vi "application.vi"() -> ()   [LabVIEW 2014, in "application.lvclass"]
uses:
  application.lvclass
  application.lvclass/application.ctl
  <vilib>/Utility/config.llb/NI_LVConfig.lvlib
panel:
  in  "Tab Control":enum32{"Main", "Settings"}(tab)
  in  "Settings":bool
  out "CMD":string caption="命令行"
  in  "file path":path=path "D:/Projects/Personal/Multi-LabVIEW-Selector/Multi-LabVIEW Selector.lvproj" caption="打开文件路径"
  in  "LabVIEW List":string(combo)
  in  "OK":bool
  in  "Cancel":bool
  in  "associate file extension":bool
  in  "System Array":string[](array[string]) caption="File Extension"
  in  "Display Time(ms)":i32 min=0 max=10000 step=100
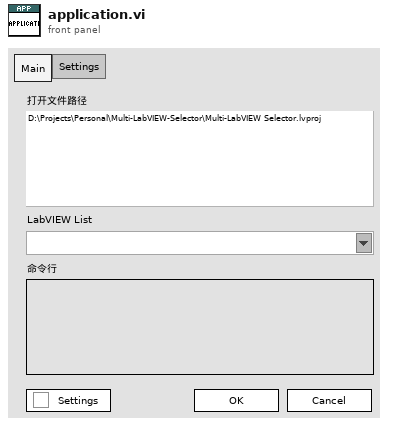
[diagram p1: front panel]
types:
  T1 = enum32{"invalid app kind", "Development System", "Run Time System", "Student Edition", "Embedded LabVIEW", "Evaluation", "Custom"}
  T2 = enum32{"Invalid", "Standard", "Closed", "Hidden", "Minimized", "Maximized"}
  T3 = cluster{"Core":cluster{"Current VI Reference":refnum<vi>, "Close Panel on Exit?":bool}, "RuntimeEngine":bool, "ConfigFilePath":path}
  T4 = cluster{"Current VI Reference":refnum<vi>, "Close Panel on Exit?":bool}
  T5 = typedef "NI_LVConfig.lvlib/Config Data RefNum.ctl" = refnum<k1>
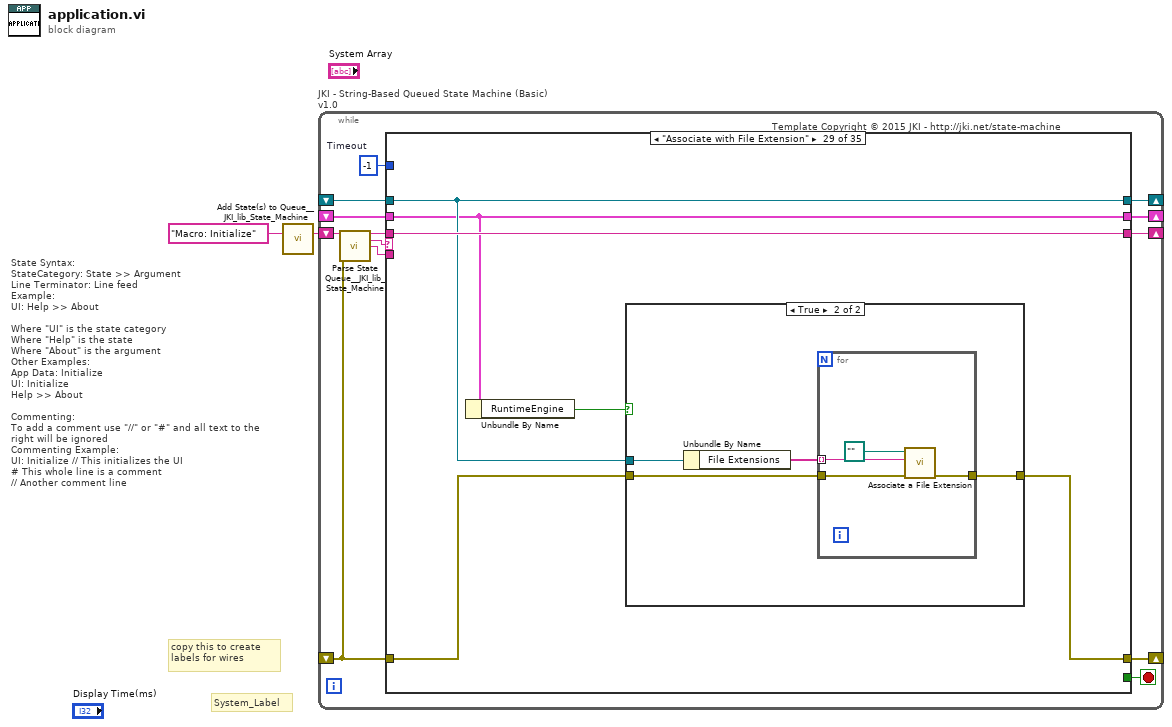
[diagram p0: block diagram]
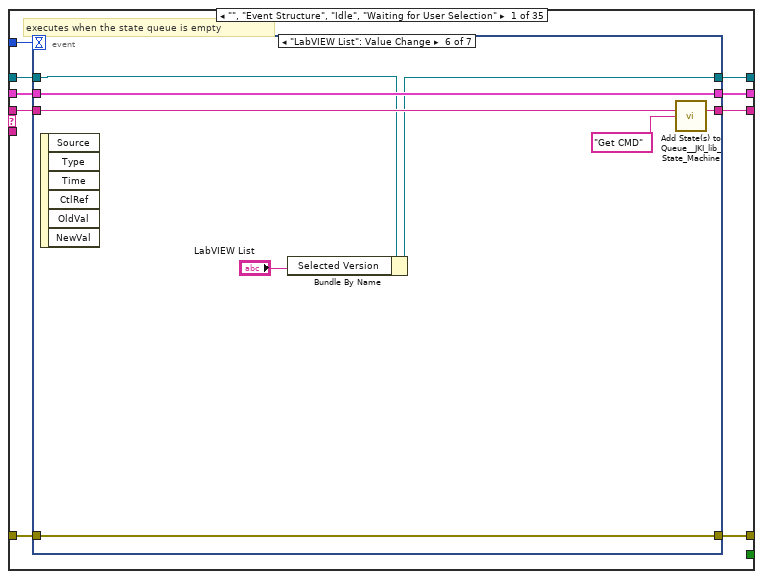
[diagram p2: hidden frame]
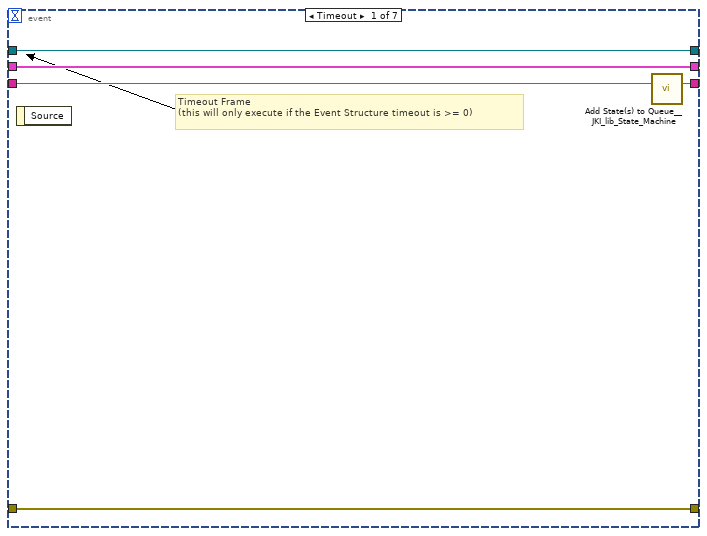
[diagram p3: hidden frame]
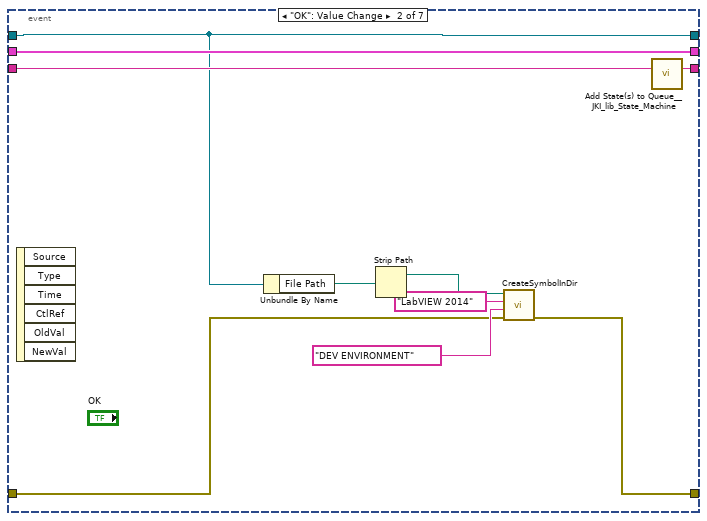
[diagram p4: hidden frame]
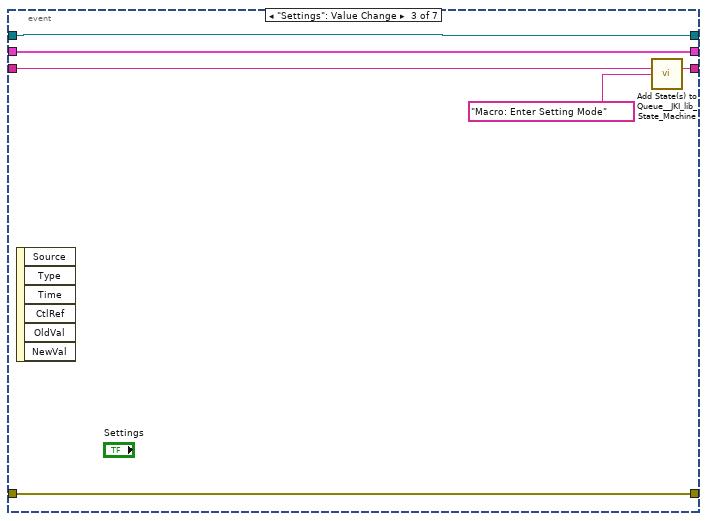
[diagram p5: hidden frame]
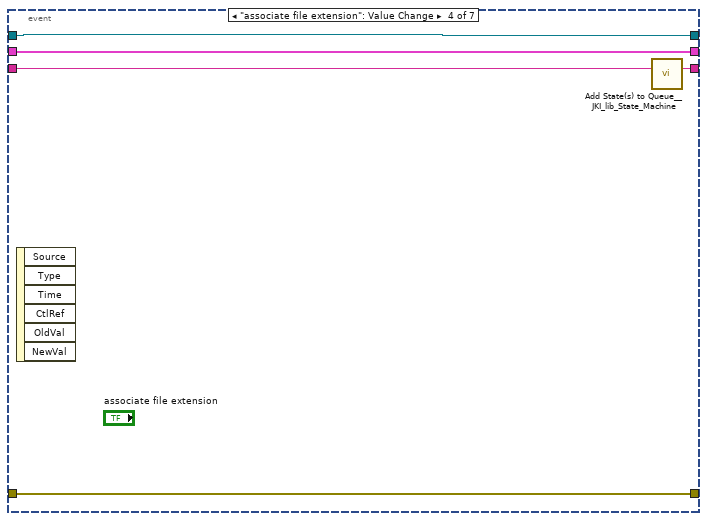
[diagram p6: hidden frame]
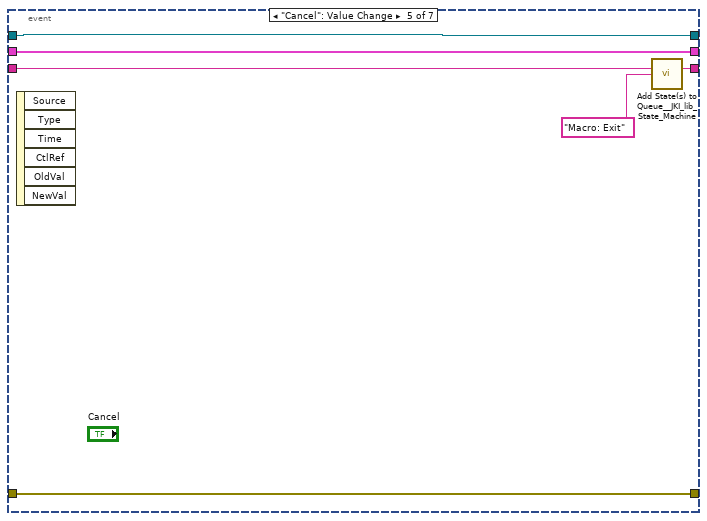
[diagram p7: hidden frame]
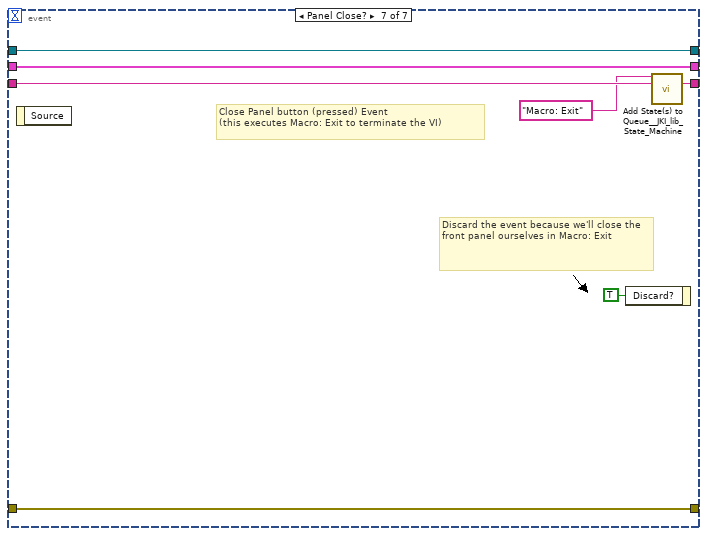
[diagram p8: hidden frame]
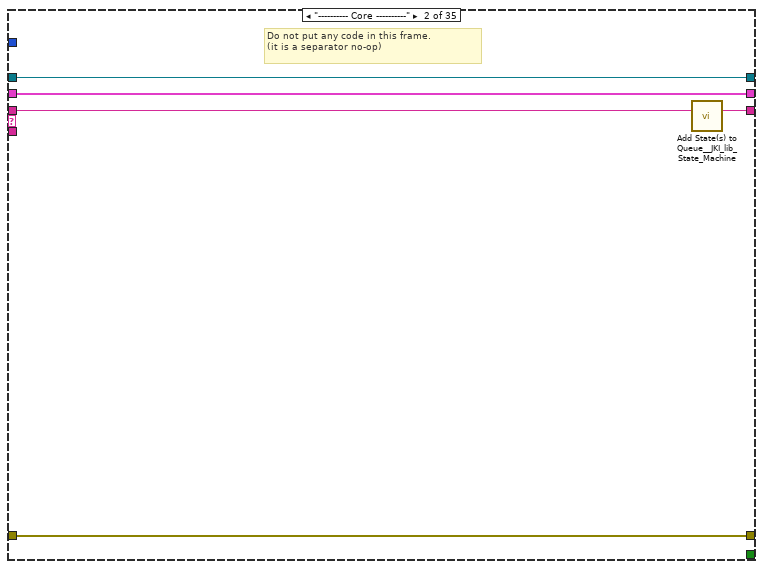
[diagram p9: hidden frame]
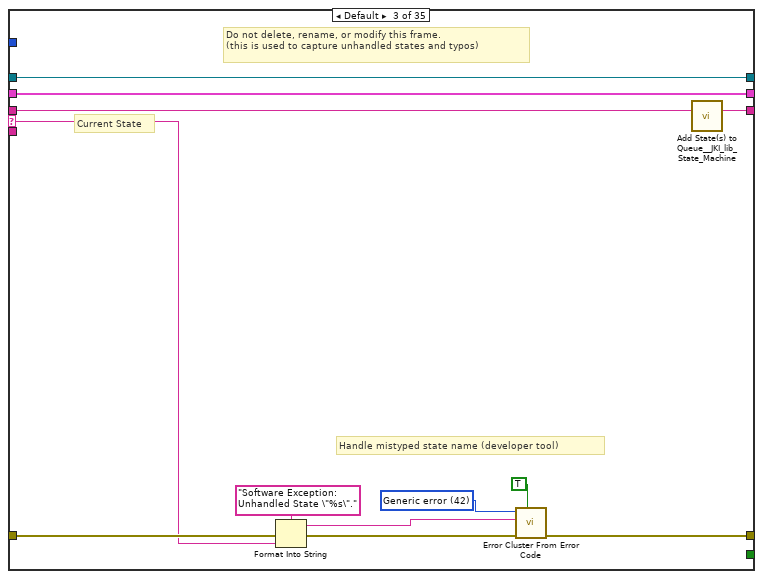
[diagram p10: hidden frame]
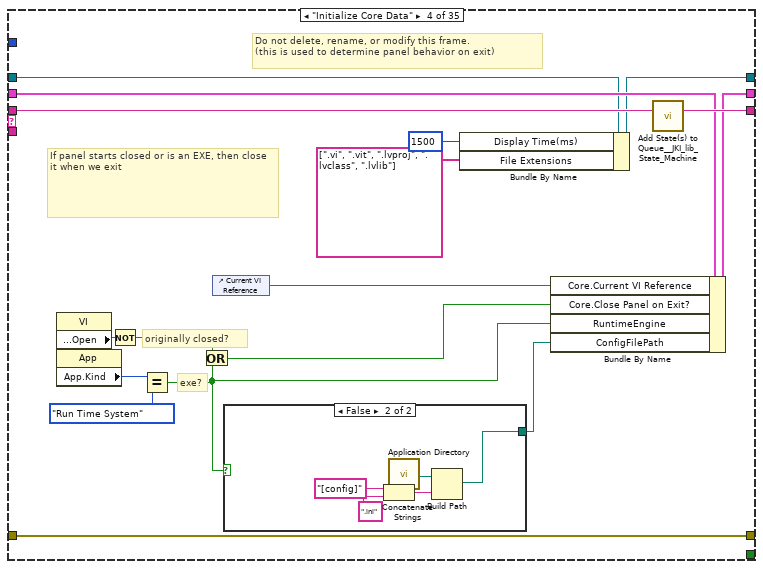
[diagram p11: hidden frame]
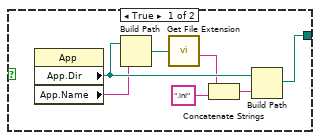
[diagram p12: hidden frame]
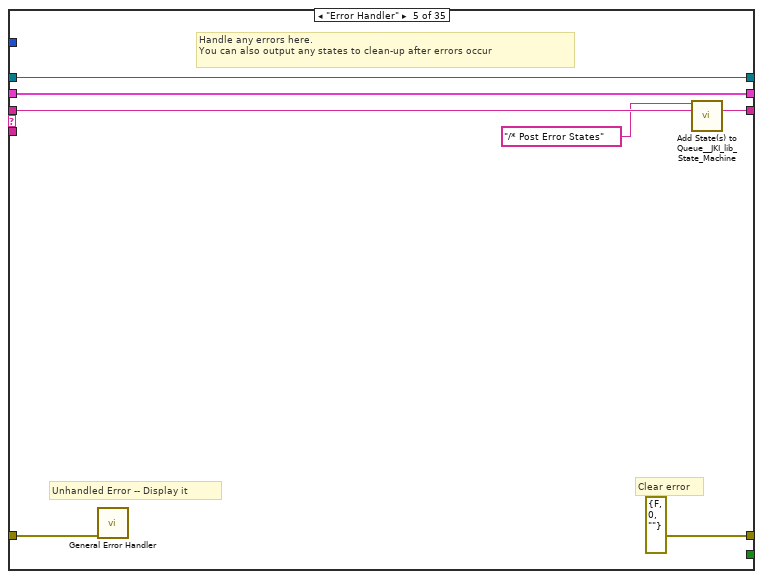
[diagram p13: hidden frame]
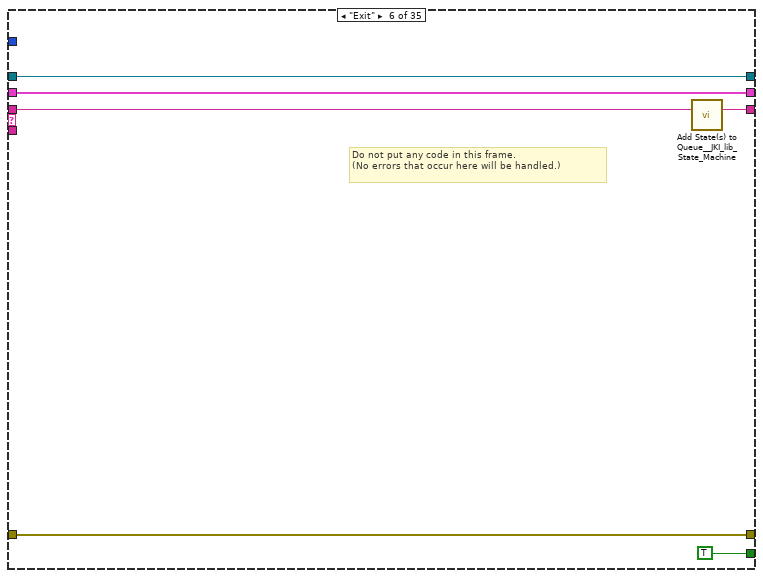
[diagram p14: hidden frame]
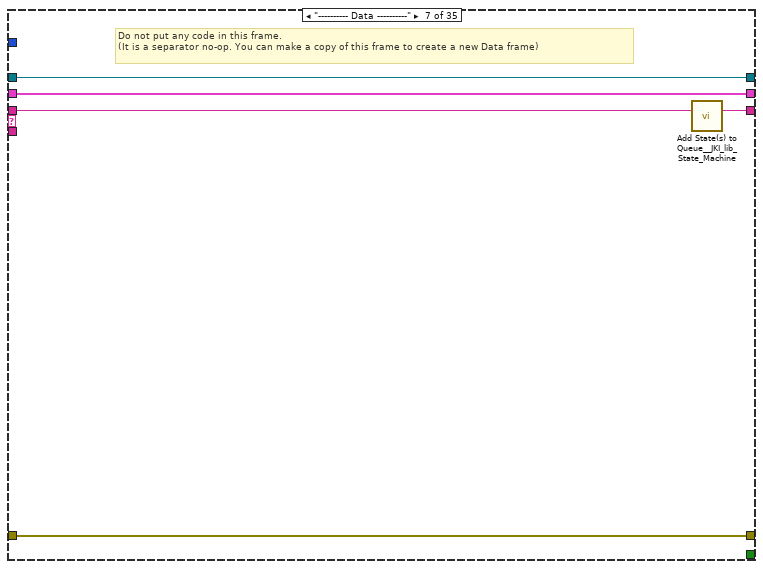
[diagram p15: hidden frame]
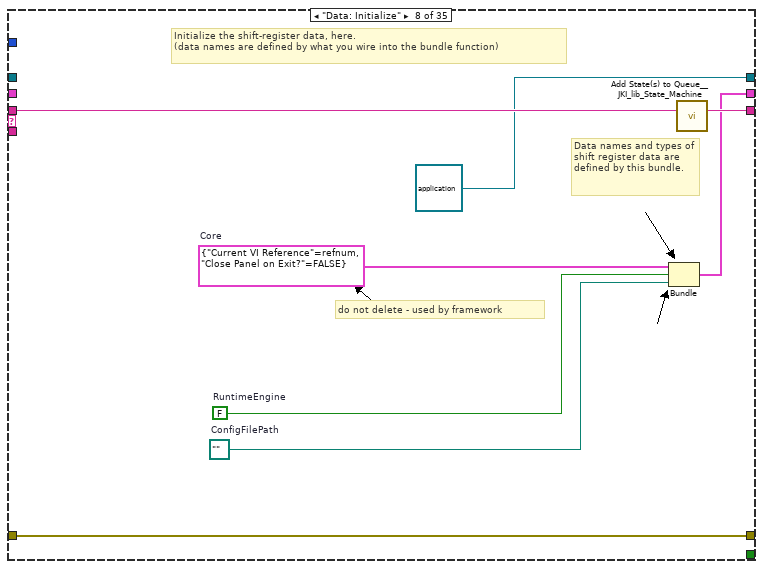
[diagram p16: hidden frame]
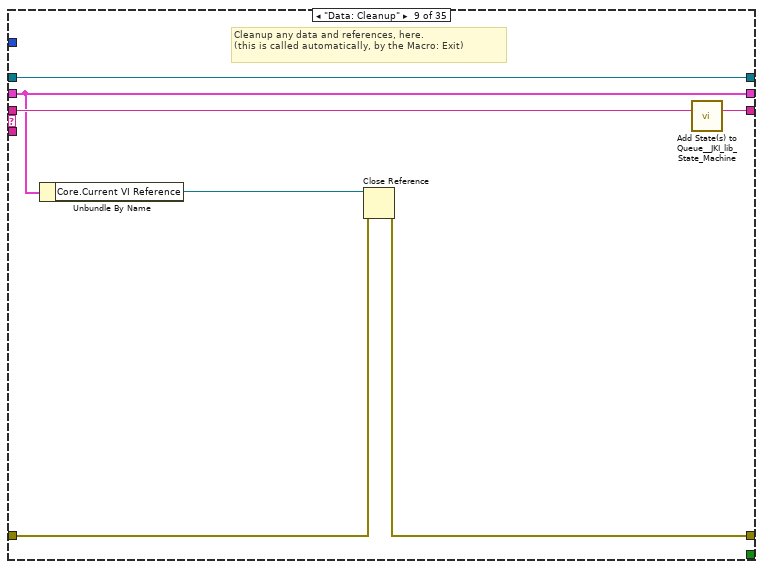
[diagram p17: hidden frame]
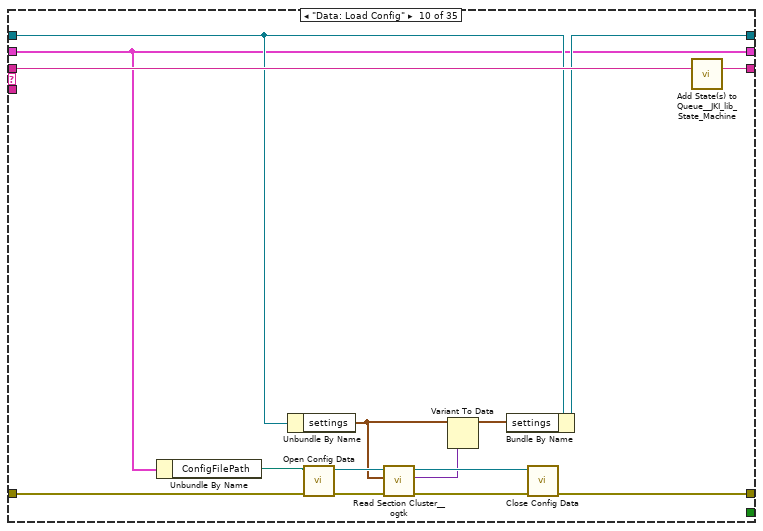
[diagram p18: hidden frame]
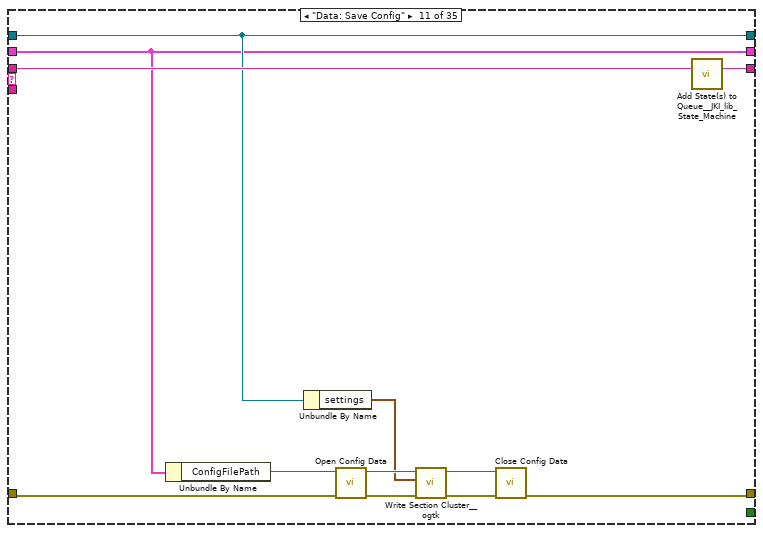
[diagram p19: hidden frame]
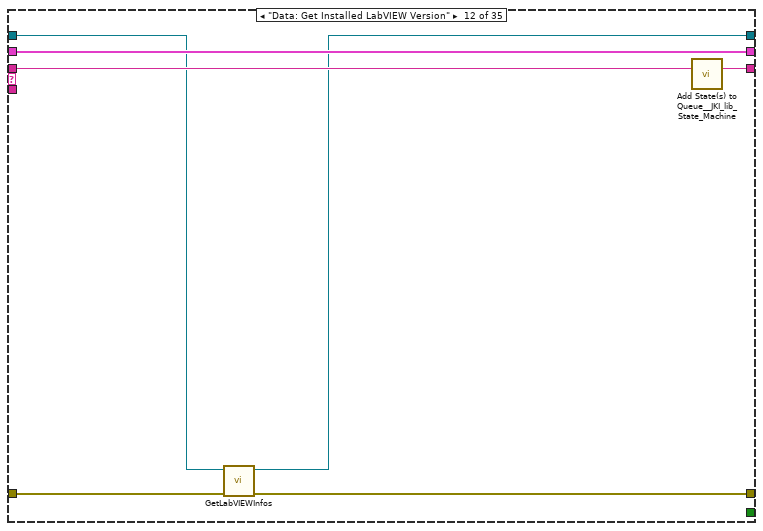
[diagram p20: hidden frame]
diagram:
  # "State Syntax:\nStateCategory: State >> Argument\nLine Terminator: Line feed\nExample:\nUI: Help >> About\n\nWhere \"UI\" is the state category\nWhere \"Help\" is the state\nWhere \"About\" is the argument\nOther Examples:\nApp Data: Initialize\nUI: Initialize\nHelp >> About\n\nCommenting:\nTo add a comment use \"//\" or \"#\" and all text to the right will be ignored\nCommenting Example:\nUI: Initialize // This initializes the UI\n# This whole line is a comment\n// Another comment line"
  # "copy this to create labels for wires"
  # "System_Label"
  n1 = call <vilib>:"Add State(s) to Queue__JKI_lib_State_Machine.vi"("State(s) in (\"\")"="Macro: Initialize") -> ("States Out"=w2:string)  [unwired: 14 in]
  n2 = while "JKI - String-Based Queued State Machine (Basic) v1.0" {
    shift-right: [w8] -> _
    shift-left: _ -> [w7]
    shift-right: [w11] -> _
    shift-left: _ -> [w5]
    shift-right: [w10] -> _
    shift-left: w2 -> [w12]
    shift-right: [w4] -> _
    shift-left: _ -> [w3]
    stop <- w9 stop-if-true
    w6 = -1  # Timeout
    # "Template Copyright © 2015 JKI - http://jki.net/state-machine"
    n3 = call <vilib>:"Parse State Queue__JKI_lib_State_Machine.vi"("State Queue"=w12, "Error In (no error)"=w5) -> ("Remaining States"=w14:string, "Current State"=w15:string, "Arguments"=w13:string)  [unwired: 11 in]
    n4 = case shown="\"Associate with File Extension\"" w15 {
      selector: w15 -> [_ _ w78 _ _ _ _ _ _ _ _ _ _ _ _ _ _ _ _ _ _ _ _ _ _ _ _ _ _ _ _ _ _ _ _]
      tunnel: w14 -> [w24 w76 w82 w105 w124 w130 w135 w143 w150 w165 w177 w184 w189 w200 w211 w223 w251 w259 w266 w273 w280 w286 w297 w303 w309 w314 w322 w325 w336 w350 w359 w383 w396 w408 w417]
      tunnel: w13 -> [_ _ _ _ _ _ _ _ _ _ _ _ _ _ w206 w217 _ _ _ w268 _ _ _ _ _ _ _ _ _ _ _ _ _ _ _]
      tunnel: w7 -> [w22 w73 w80 w97 w121 w128 w132 _ w145 w152 w166 w182 w186 w198 w209 w219 w248 w256 w263 w270 w277 w283 w294 w300 w306 w311 w320 w326 w332 w347 w355 w385 w398 w410 w419]
      tunnel: [w21 w74 w84 w102 errorcluster {"status"=FALSE, "code"=0, "source"=""} ("error out") w127 w133 w140 w146 w157 w170 w180 w187 w196 w207 w220 w249 w257 w264 w271 w278 w284 w295 w301 w307 w312 w318 w323 w334 w348 w361 w373 w386 w399 w416] -> w11
      tunnel: w5 -> [w20 w74 w83 w102 w120 w127 w133 w140 w147 w158 w169 w181 w187 w194 w208 w221 w249 w257 w264 w271 w278 w284 w295 w301 w307 w312 w319 w324 w335 w348 w362 w374 w387 w400 w416]
      tunnel: [w23 w75 w81 w104 w123 w129 w134 w142 w149 w164 w176 w183 w188 w199 w210 w222 w250 w258 w265 w272 w279 w285 w296 w302 w308 w313 w321 w325 w336 w349 w360 w384 w397 w409 w418] -> w10
      tunnel: [_ _ _ _ _ TRUE _ _ _ _ _ _ _ _ _ _ _ _ _ _ _ _ _ _ _ _ _ _ _ _ _ _ _ _ _] -> w9
      tunnel: [w19 w73 w80 w103 w121 w128 w132 w141 w145 w152 w166 w182 w186 w198 w209 w219 w248 w256 w263 w270 w277 w283 w294 w300 w306 w311 w320 w326 w332 w347 w355 w385 w398 w410 w419] -> w8
      tunnel: w6 -> [w18 _ _ _ _ _ _ _ _ _ _ _ _ _ _ _ _ _ _ _ _ _ _ _ _ _ _ _ _ _ _ _ _ _ _]
      tunnel: [w16 w72 w77 w93 w118 w125 w131 refnum<class "application.lvclass"> refnum ("application.lvclass") w144 w156 w168 w178 w185 w197 w205 w216 w247 w253 w262 w269 w276 w281 w287 w299 w305 w310 w316 w327 w333 w346 w358 w375 w388 w401 w411] -> w4
      tunnel: w3 -> [w17 w72 w77 w94 w118 w125 w131 _ w144 w163 w168 w179 w185 w197 w205 w216 w247 w253 w262 w269 w276 w281 w287 w299 w305 w310 w317 w327 w333 w346 w363 w376 w389 w401 w412]
      frame "", "Event Structure", "Idle", "Waiting for User Selection" {
        # "executes when the state queue is empty"
        n5 = event shown="[5] \"LabVIEW List\": Value Change" {
          selector: _ -> [_ _ _ _ _ _ _]
          dyn-events: _ -> [_ _ _ _ _ _ _]
          timeout: w18 -> [_ _ _ _ _ _ _]
          tunnel: w24 -> [w29 w39 w45 w50 w56 w64 w71]
          tunnel: [w28 w38 w44 w49 w55 w63 w70] -> w23
          tunnel: w22 -> [w26 w37 w42 w47 w53 w61 w68]
          tunnel: [w27 w31 w43 w48 w54 w62 w69] -> w21
          tunnel: w20 -> [w27 w32 w43 w48 w54 w62 w69]
          tunnel: [w26 w37 w42 w47 w53 w61 w68] -> w19
          tunnel: w17 -> [w25 w33 w41 w46 w52 w60 w65]
          tunnel: [w25 w33 w41 w46 w52 w58 w65] -> w16
          event Timeout {
            # "Timeout Frame\n(this will only execute if the Event Structure timeout is >= 0)"
            n6 = event-data() -> ()  [unwired: 1 in, 1 out]
            n7 = call <vilib>:"Add State(s) to Queue__JKI_lib_State_Machine.vi"("State(s) in (\"\")"=w29) -> ("States Out"=w28:string)  [unwired: 14 in]
          }
          event "OK": Value Change {
            n8 = event-data() -> ()  [unwired: 1 in, 6 out]
            n9 = Unbundle By Name(w33) -> ("File Path"=w36:path)
            n10 = Strip Path(path=w36) -> (stripped path=w35:path)  [unwired: 1 out]
            n11 = call "CreateSymbolInDir.vi"("error in"=w32, "prefix"="DEV ENVIRONMENT", "Name"="LabVIEW 2014", "Path"=w35) -> ("error out"=w31:errorcluster)  [unwired: 6 in, 1 out]
            n12 = call <vilib>:"Add State(s) to Queue__JKI_lib_State_Machine.vi"("State(s) in (\"\")"=w39) -> ("States Out"=w38:string)  [unwired: 14 in]
          }
          event "Settings": Value Change {
            n13 = event-data() -> ()  [unwired: 1 in, 6 out]
            n14 = call <vilib>:"Add State(s) to Queue__JKI_lib_State_Machine.vi"("State(s) in (\"\")"=w45, "State(s) at Back (\"\")"="Macro: Enter Setting Mode" ("State(s) at Back (\"\")")) -> ("States Out"=w44:string)  [unwired: 13 in]
          }
          event "associate file extension": Value Change {
            n15 = event-data() -> ()  [unwired: 1 in, 6 out]
            n16 = call <vilib>:"Add State(s) to Queue__JKI_lib_State_Machine.vi"("State(s) in (\"\")"=w50) -> ("States Out"=w49:string)  [unwired: 14 in]
          }
          event "Cancel": Value Change {
            n17 = event-data() -> ()  [unwired: 1 in, 6 out]
            n18 = call <vilib>:"Add State(s) to Queue__JKI_lib_State_Machine.vi"("State(s) in (\"\")"=w56, "State(s) at Back (\"\")"="Macro: Exit" ("State(s) at Back (\"\")")) -> ("States Out"=w55:string)  [unwired: 13 in]
          }
          event "LabVIEW List": Value Change {
            n19 = event-data() -> ()  [unwired: 1 in, 6 out]
            n20 = Bundle By Name(cluster=w60, "Selected Version"="LabVIEW List") -> (w58:refnum<class "application.lvclass">)
            n21 = call <vilib>:"Add State(s) to Queue__JKI_lib_State_Machine.vi"("State(s) in (\"\")"=w64, "State(s) at Back (\"\")"="Get CMD" ("State(s) at Back (\"\")")) -> ("States Out"=w63:string)  [unwired: 13 in]
          }
          event Panel Close? {
            # "Discard the event because we'll close the front panel ourselves in Macro: Exit"
            # "Close Panel button (pressed) Event\n(this executes Macro: Exit to terminate the VI)"
            n22 = event-data() -> ()  [unwired: 1 in, 1 out]
            n23 = event-data("Discard?"=TRUE) -> ()  [unwired: 1 in, 1 out]
            n24 = call <vilib>:"Add State(s) to Queue__JKI_lib_State_Machine.vi"("State(s) in Front (\"\")"="Macro: Exit", "State(s) in (\"\")"=w71) -> ("States Out"=w70:string)  [unwired: 13 in]
          }
        }
      }
      frame "---------- Core ----------" {
        # "Do not put any code in this frame.\n(it is a separator no-op)"
        n25 = call <vilib>:"Add State(s) to Queue__JKI_lib_State_Machine.vi"("State(s) in (\"\")"=w76) -> ("States Out"=w75:string)  [unwired: 14 in]
      }
      frame Default {
        w87 = 42 items=["No error", "Argument error", "Memory is full", "Out of zone", "End of file", "File already open", "Generic file I/O error", "File not found", "File permission error", "Disk is full", "Duplicate path", "Too many files open", "System feature not enabled", "Resource file not found", "Cannot add resource", "Resource not found", "Image not found", "Image memory error", "Pen does not exist", "Config type invalid", "Config token not found", "Config parse error", "Config memory error", "Bad external code format", "Bad external code offset", "External code not present", "Null window", "Destroy window error", "Null menu", "Print aborted", "Bad print record", "Print driver error", "Windows error during printing", "Memory error during printing", "Print dialog error", "Generic print error", "Invalid device refnum", "Device not found", "Device parameter error", "Device unit error", "Cannot open device", "Device call aborted", "Generic error", "Cancelled by user", "Object ID too low", "Object ID too high", "Object not in heap", "Unknown heap", "Unknown object (invalid DefProc)", "Unknown object (DefProc not in table)", "Message out of range", "Invalid (null) method", "Unknown message", "Manager call not supported", "Bad address", "Network operation in progress", "Network operation timed out", "Connection is busy", "Network attribute not supported", "Network error", "Address in use", "System out of memory", "Connection aborted", "Connection refused", "Not connected", "Already connected", "Connection closed", "Initialization error (interapplication manager)", "Bad occurrence", "Wait on unbound occurrence handler", "Occurrence queue overflow", "Datalog type conflict", "Unused", "Unrecognized type (interapplication manager)", "Memory corrupt", "Failed to make temporary DLL", "Old CIN version", "Drag socket not found", "Failed to load drop-object", "Failed to register OLE object", "Failed to release OLE object", "Format specifier type mismatch", "Unknown format specifier", "Too few format specifiers", "Too many format specifiers", "Scan failed", "Newer CIN version", "Error converting to variant", "Runtime menu error", "Password tampered", "Variant attribute not found", "Incompatible variant data type", "Event data is not available", "Event Store is not present", "Occurrence is not found", "Event Queue is not created", "Event info is not available", "Refnum passed is NULL", "Error retrieving Class GUID", "Error retrieving CoClass GUID", "Error retrieving TypeLib GUID.", "Bad built application magic bytes.", "Specific driver is different from the specific driver associated with the Logical Name.", "There is no session opened to the class driver.", "Max Error", "MAX - Error with config objects", "MAX - Error loading configuration", "MAX - Group not supported"]
        # "Current State"
        # "Do not delete, rename, or modify this frame.\n(this is used to capture unhandled states and typos)"
        # "Handle mistyped state name (developer tool)"
        n26 = Format Into String(format string="Software Exception: Unhandled State \"%s\"." ("message"), error in=w83, w78) -> (resulting string=w86:string, error out=w85:errorcluster)  [unwired: 1 in]
        n27 = call <vilib>:"Error Cluster From Error Code.vi"("show call chain? (False)"=TRUE, "error in (no error)"=w85, "error message (\"\")"=w86, "error code (0)"=w87) -> ("error out"=w84:errorcluster)  [unwired: 5 in]
        n28 = call <vilib>:"Add State(s) to Queue__JKI_lib_State_Machine.vi"("State(s) in (\"\")"=w82) -> ("States Out"=w81:string)  [unwired: 14 in]
      }
      frame "Initialize Core Data" {
        # "Do not delete, rename, or modify this frame.\n(this is used to determine panel behavior on exit)"
        # "originally closed?"
        # "exe?"
        # "If panel starts closed or is an EXE, then close it when we exit"
        n29 = property class="VI"() -> ("Front Panel.Open"=w101:bool)  [unwired: 2 in, 2 out]
        n30 = property class="App"() -> ("App.Kind"=w100:T1)  [unwired: 2 in, 2 out]
        n31 = Not(x=w101) -> (.not. x?=w98:bool)
        n32 = Equal?(x=w100, y=T1."Run Time System" ("Application:Kind")) -> (x = y?=w89:bool)
        n33 = Or(x=w98, y=w89) -> (x .or. y?=w96:bool)
        n34 = control-ref of="Current VI Reference"() -> (w95:refnum<vi>)
        n35 = case shown="False" w89 {
          tunnel: [w110 w114] -> w90
          frame True {
            n36 = property class="App"() -> ("App.Dir"=w109:path, "App.Name"=w108:string)  [unwired: 2 in, 2 out]
            n37 = Build Path(base path=w109, name or relative path=w108) -> (appended path=w107:path)
            n38 = call <vilib>:"Get File Extension.vi"("file"=w107) -> ("filename without extension"=w106:string)  [unwired: 7 in, 3 out]
            n39 = Concatenate Strings(w106, ".ini" ("Application:Name")) -> (w111:string)
            n40 = Build Path(base path=w109, name or relative path=w111) -> (appended path=w110:path)
          }
          frame False {
            n41 = Concatenate Strings("[config]" ("string"), ".ini" ("Application:Name")) -> (w115:string)
            n42 = call <vilib>:"Application Directory.vi"() -> ("Application Directory"=w116:path)
            n43 = Build Path(base path=w116, name or relative path=w115) -> (appended path=w114:path)
          }
        }
        n44 = Bundle By Name(cluster=w94, "Display Time(ms)"=1500 ("settings.Display Time(ms)"), "File Extensions"=string[] [".vi", ".vit", ".lvproj", ".lvclass", ".lvlib"]) -> (w93:refnum<class "application.lvclass">)
        n45 = Bundle By Name(cluster=w97, "Core.Current VI Reference"=w95, "Core.Close Panel on Exit?"=w96, "RuntimeEngine"=w89, "ConfigFilePath"=w90) -> (w103:T3)
        n46 = call <vilib>:"Add State(s) to Queue__JKI_lib_State_Machine.vi"("State(s) in (\"\")"=w105) -> ("States Out"=w104:string)  [unwired: 14 in]
      }
      frame "Error Handler" {
        # "Unhandled Error -- Display it"
        # "Handle any errors here.\nYou can also output any states to clean-up after errors occur"
        # "Clear error"
        n47 = call <vilib>:"General Error Handler.vi"("error in (no error)"=w120) -> ()  [unwired: 10 in, 5 out]
        n48 = call <vilib>:"Add State(s) to Queue__JKI_lib_State_Machine.vi"("State(s) in Front (\"\")"="/* Post Error States", "State(s) in (\"\")"=w124) -> ("States Out"=w123:string)  [unwired: 13 in]
      }
      frame "Exit" {
        # "Do not put any code in this frame.\n(No errors that occur here will be handled.)"
        n49 = call <vilib>:"Add State(s) to Queue__JKI_lib_State_Machine.vi"("State(s) in (\"\")"=w130) -> ("States Out"=w129:string)  [unwired: 14 in]
      }
      frame "---------- Data ----------" {
        # "Do not put any code in this frame.\n(It is a separator no-op. You can make a copy of this frame to create a new Data frame)"
        n50 = call <vilib>:"Add State(s) to Queue__JKI_lib_State_Machine.vi"("State(s) in (\"\")"=w135) -> ("States Out"=w134:string)  [unwired: 14 in]
      }
      frame "Data: Initialize" {
        w137 = T4 {"Current VI Reference"=refnum, "Close Panel on Exit?"=FALSE}  # Core
        w139 = FALSE  # RuntimeEngine
        w138 = path ""  # ConfigFilePath
        # "do not delete - used by framework"
        # "Data names and types of shift register data are defined by this bundle."
        # "Initialize the shift-register data, here.\n(data names are defined by what you wire into the bundle function)"
        n51 = Bundle("Core"=w137, "RuntimeEngine"=w139, "ConfigFilePath"=w138) -> (w141:T3)  [unwired: 1 in]
        n52 = call <vilib>:"Add State(s) to Queue__JKI_lib_State_Machine.vi"("State(s) in (\"\")"=w143) -> ("States Out"=w142:string)  [unwired: 14 in]
      }
      frame "Data: Cleanup" {
        # "Cleanup any data and references, here.\n(this is called automatically, by the Macro: Exit)"
        n53 = Unbundle By Name(w145) -> ("Core.Current VI Reference"=w148:refnum<vi>)
        n54 = Close Reference(reference=w148, error in (no error)=w147) -> (error out=w146:errorcluster)
        n55 = call <vilib>:"Add State(s) to Queue__JKI_lib_State_Machine.vi"("State(s) in (\"\")"=w150) -> ("States Out"=w149:string)  [unwired: 14 in]
      }
      frame "Data: Load Config" {
        n56 = Unbundle By Name(w152) -> ("ConfigFilePath"=w151:path)
        n57 = Unbundle By Name(w163) -> ("settings"=w153:cluster{"Display Time(ms)":i32})
        n58 = call <vilib>:"Open Config Data.vi"("error in (no error)"=w158, "configuration file path"=w151) -> ("error out"=w161:errorcluster, "refnum"=w162:T5)  [unwired: 7 in, 1 out]
        n59 = call <userlib>:"Read Section Cluster__ogtk.vi"("error in (no error)"=w161, "Section Formatted Cluster Type"=w153, "refnum"=w162) -> ("error out"=w159:errorcluster, "Section Formatted Cluster"=w154:variant, "dup refnum"=w160:T5)  [unwired: 4 in, 2 out]
        n60 = Variant To Data(type=w153, Variant=w154) -> (data=w155:cluster{"Display Time(ms)":i32})  [unwired: 1 in, 1 out]
        n61 = Bundle By Name(cluster=w163, "settings"=w155) -> (w156:refnum<class "application.lvclass">)
        n62 = call <vilib>:"Close Config Data.vi"("error in (no error)"=w159, "refnum"=w160) -> ("error out"=w157:errorcluster)  [unwired: 8 in, 1 out]
        n63 = call <vilib>:"Add State(s) to Queue__JKI_lib_State_Machine.vi"("State(s) in (\"\")"=w165) -> ("States Out"=w164:string)  [unwired: 14 in]
      }
      frame "Data: Save Config" {
        n64 = Unbundle By Name(w166) -> ("ConfigFilePath"=w167:path)
        n65 = Unbundle By Name(w168) -> ("settings"=w171:cluster{"Display Time(ms)":i32})
        n66 = call <vilib>:"Open Config Data.vi"("error in (no error)"=w169, "configuration file path"=w167) -> ("error out"=w174:errorcluster, "refnum"=w175:T5)  [unwired: 7 in, 1 out]
        n67 = call <userlib>:"Write Section Cluster__ogtk.vi"("error in (no error)"=w174, "Section Formatted Cluster"=w171, "refnum"=w175) -> ("error out"=w172:errorcluster, "dup refnum"=w173:T5)  [unwired: 7 in]
        n68 = call <vilib>:"Close Config Data.vi"("error in (no error)"=w172, "refnum"=w173) -> ("error out"=w170:errorcluster)  [unwired: 8 in, 1 out]
        n69 = call <vilib>:"Add State(s) to Queue__JKI_lib_State_Machine.vi"("State(s) in (\"\")"=w177) -> ("States Out"=w176:string)  [unwired: 14 in]
      }
      frame "Data: Get Installed LabVIEW Version" {
        n70 = call "GetLabVIEWInfos.vi"("error in (no error)"=w181, "application.lvclass"=w179) -> ("error out"=w180:errorcluster, "application.lvclass (dup)"=w178:refnum<class "application.lvclass">)  [unwired: 8 in]
        n71 = call <vilib>:"Add State(s) to Queue__JKI_lib_State_Machine.vi"("State(s) in (\"\")"=w184) -> ("States Out"=w183:string)  [unwired: 14 in]
      }
      frame "---------- UI ----------" {
        # "Do not put any code in this frame.\n(It is a separator no-op. You can make a copy of this frame to create a new UI frame)"
        n72 = call <vilib>:"Add State(s) to Queue__JKI_lib_State_Machine.vi"("State(s) in (\"\")"=w189) -> ("States Out"=w188:string)  [unwired: 14 in]
      }
      frame "UI: Initialize" {
        # "Initialize the User Interface, here.\n(this is called automatically, by the Macro: Init)"
        n73 = disable-structure shown="Default" {
          disable-tunnel: [FALSE ("Tabs Visible?") TRUE ("Tabs Visible?")] -> w192
          disable-tunnel: [w201 w203] -> w191
          disable-tunnel: [w201 w203] -> w190
          frame condition #0 {
            w201 = u32 16777216
          }
          frame condition #1 (active) {
            w203 = u32 16777216
          }
        }
        n74 = property on="Tab Control" class="TabCtl (strict)"(error in=w194, "Tabs Visible?"=w192, "BG Color"=w191, "FG Color"=w190) -> (error out=w193:errorcluster)  [unwired: 1 in, 1 out]
        n75 = call <userlib>:"Fit VI window to Content__ogtk.vi"("error in (no error)"=w193, "border spacing (2 px)"=0) -> ("error out"=w196:errorcluster)  [unwired: 4 in, 1 out]
        n76 = call <vilib>:"Add State(s) to Queue__JKI_lib_State_Machine.vi"("State(s) in (\"\")"=w200) -> ("States Out"=w199:string)  [unwired: 14 in]
      }
      frame "UI: Cursor Set" {
        # "Argument"
        # "Set and Unset Cursor Busy.\n(Usage: \"UI: Cursor Set >> Busy|Idle\")"
        n77 = case shown="\"Idle\", Default" w206 {
          tunnel: w208 -> [w213 w215]
          tunnel: [w212 w214] -> w207
          frame "Idle", Default {
            n78 = call <vilib>:"Unset Busy.vi"("error in (no error)"=w213) -> ("error out"=w212:errorcluster)  [unwired: 10 in]
          }
          frame "Busy" {
            n79 = call <vilib>:"Set Busy.vi"("error in (no error)"=w215) -> ("error out"=w214:errorcluster)  [unwired: 9 in, 1 out]
          }
        }
        n80 = call <vilib>:"Add State(s) to Queue__JKI_lib_State_Machine.vi"("State(s) in (\"\")"=w211) -> ("States Out"=w210:string)  [unwired: 14 in]
      }
      frame "UI: Front Panel State" {
        # "Argument"
        # "Set Front Panel Open or Closed\n(Usage: \"UI: Front Panel State >> Open|Close\")"
        n81 = Unbundle By Name(w219) -> ("Core.Current VI Reference"=w218:refnum<vi>)
        n82 = case shown="\"Open\", Default" w217 {
          tunnel: w221 -> [w227 w240]
          tunnel: [w229 w241] -> w220
          tunnel: w218 -> [w228 w238]
          frame "Open", Default {
            n83 = property class="VI"(reference=w228, error in=w227) -> (reference out=w225:refnum<vi>, error out=w226:errorcluster, "Front Panel.Open"=w224:bool)
            n84 = case shown="False" w224 {
              tunnel: [w232 w235] -> w229
              tunnel: w226 -> [w231 w235]
              tunnel: w225 -> [w230 _]
              frame False {
                n85 = invoke class="VI" method="FP.Open"(reference=w230, error in=w231, "Activate"=TRUE, "State"=T2."Standard") -> (error out=w232:errorcluster)  [unwired: 1 in, 4 out]
              }
              frame True {
              }
            }
          }
          frame "Close" {
            n86 = property class="VI"(reference=w238, error in=w240) -> (reference out=w237:refnum<vi>, error out=w239:errorcluster, "Front Panel.Open"=w236:bool)
            n87 = case shown="True" w236 {
              tunnel: [w242 w245] -> w241
              tunnel: w239 -> [w242 w244]
              tunnel: w237 -> [_ w243]
              frame False {
              }
              frame True {
                n88 = invoke class="VI" method="FP.Close"(reference=w243, error in=w244) -> (error out=w245:errorcluster)  [unwired: 1 in, 2 out]
              }
            }
          }
        }
        n89 = call <vilib>:"Add State(s) to Queue__JKI_lib_State_Machine.vi"("State(s) in (\"\")"=w223) -> ("States Out"=w222:string)  [unwired: 14 in]
      }
      frame "UI: Display CMD" {
        n90 = Unbundle By Name(w247) -> ("CMD line"=→"CMD":string)
        n91 = call <vilib>:"Add State(s) to Queue__JKI_lib_State_Machine.vi"("State(s) in (\"\")"=w251) -> ("States Out"=w250:string)  [unwired: 14 in]
      }
      frame "UI: Display LabVIEW Information" {
        n92 = Unbundle By Name(w253) -> ("Version List"=w255:string[], "Selected Version"=w254:string)
        n93 = control-ref of="LabVIEW List"() -> (w252:refnum<vi>)
        n94 = property on="Property Node" class="CmbBox"(reference=w252, "Strings[]"=w255, "Value"=w254) -> ()  [unwired: 1 in, 2 out]
        n95 = call <vilib>:"Add State(s) to Queue__JKI_lib_State_Machine.vi"("State(s) in (\"\")"=w259) -> ("States Out"=w258:string)  [unwired: 14 in]
      }
      frame "UI: Display Settings" {
        n96 = Unbundle By Name(w262) -> ("Display Time(ms)"=w261:i32, "File Extensions"=w260:string[])
        n97 = local write "Display Time(ms)"(w261) -> ()
        n98 = local write "System Array"(w260) -> ()
        n99 = call <vilib>:"Add State(s) to Queue__JKI_lib_State_Machine.vi"("State(s) in (\"\")"=w266) -> ("States Out"=w265:string)  [unwired: 14 in]
      }
      frame "UI: Switch Page" {
        n100 = case shown="\"Settings\"" w268 {
          tunnel: [enum32{"Main", "Settings"}."Settings" ("Tab Control") enum32{"Main", "Settings"}."Main" ("Tab Control")] -> w267
          frame "Settings" {
          }
          frame Default {
          }
        }
        n101 = local write "Tab Control"(w267) -> ()
        n102 = call <vilib>:"Add State(s) to Queue__JKI_lib_State_Machine.vi"("State(s) in (\"\")"=w273) -> ("States Out"=w272:string)  [unwired: 14 in]
      }
      frame "---------- Macro ----------" {
        # "Do not put any code in this frame.\n(It is a separator no-op. You can make a copy of this frame to create a new Macro frame)"
        n103 = call <vilib>:"Add State(s) to Queue__JKI_lib_State_Machine.vi"("State(s) in (\"\")"=w280) -> ("States Out"=w279:string)  [unwired: 14 in]
      }
      frame "Macro: Initialize" {
        # "Initialization Macro\n(This is called once, when the VI starts)"
        n104 = call <vilib>:"Add State(s) to Queue__JKI_lib_State_Machine.vi"("State(s) in Front (\"\")"="Data: Initialize\nInitialize Core Data\nData: Load Config\nUI: Initialize\nUI: Display LabVIEW Information\nUI: Display Settings\nUI: Front Panel State >> Open\nGet Opened File Name", "State(s) in (\"\")"=w286) -> ("States Out"=w285:string)  [unwired: 13 in]
      }
      frame "Macro: Exit" {
        # "Exit Macro\n(This is called once, when the VI exits)"
        n105 = Unbundle By Name(w294) -> ("Core.Close Panel on Exit?"=w293:bool)
        n106 = Select(t="UI: Front Panel State >> Close", s=w293, f="") -> (s? t:f=w290:string)
        n107 = call <vilib>:"Add State(s) to Queue__JKI_lib_State_Machine.vi"("State(s) in (\"\")"=w290, "State(s) at Back (\"\")"="Data: Save Config\nData: Cleanup\nExit") -> ("States Out"=w288:string)  [unwired: 13 in]
        n108 = call <vilib>:"Add State(s) to Queue__JKI_lib_State_Machine.vi"("State(s) in Front (\"\")"=w288, "State(s) in (\"\")"=w297) -> ("States Out"=w296:string)  [unwired: 13 in]
      }
      frame "Macro: Enter Setting Mode" {
        n109 = call <vilib>:"Add State(s) to Queue__JKI_lib_State_Machine.vi"("State(s) in Front (\"\")"="UI: Switch Page >> Settings" ("State(s) in Front (\"\")"), "State(s) in (\"\")"=w303) -> ("States Out"=w302:string)  [unwired: 13 in]
      }
      frame "Macro: Enter Normal Mode" {
        n110 = call <vilib>:"Add State(s) to Queue__JKI_lib_State_Machine.vi"("State(s) in Front (\"\")"="UI: Switch Page >> Normal" ("State(s) in Front (\"\")"), "State(s) in (\"\")"=w309) -> ("States Out"=w308:string)  [unwired: 13 in]
      }
      frame "---------- State Machine ----------" {
        n111 = call <vilib>:"Add State(s) to Queue__JKI_lib_State_Machine.vi"("State(s) in (\"\")"=w314) -> ("States Out"=w313:string)  [unwired: 14 in]
      }
      frame "Get CMD" {
        n112 = call "GetCMDLine.vi"("error in (no error)"=w319, "application in"=w317) -> ("error out"=w318:errorcluster, "application out"=w316:refnum<class "application.lvclass">)  [unwired: 8 in]
        n113 = call <vilib>:"Add State(s) to Queue__JKI_lib_State_Machine.vi"("State(s) in Front (\"\")"="UI: Display CMD" ("State(s) in Front (\"\")"), "State(s) in (\"\")"=w322) -> ("States Out"=w321:string)  [unwired: 13 in]
      }
      frame "Excute CMD" {
        n114 = Unbundle By Name(w327) -> ("CMD line"=w328:string)
        n115 = call <vilib>:"System Exec.vi"("run minimized? (F)"=TRUE, "wait until completion? (T)"=FALSE, "error in (no error)"=w324, "command line"=w328) -> ("error out"=w323:errorcluster)  [unwired: 4 in, 3 out]
      }
      frame "Associate with File Extension" {
        n116 = Unbundle By Name(w332) -> ("RuntimeEngine"=w331:bool)
        n117 = case shown="True" w331 {
          tunnel: w335 -> [w337 w341]
          tunnel: [w337 w340] -> w334
          tunnel: w333 -> [_ w339]
          frame False {
          }
          frame True {
            n118 = Unbundle By Name(w339) -> ("File Extensions"=w338:string[])
            n119 = for {
              tunnel: w341 -> [w345]
              tunnel: [w344] -> w340
              tunnel: w338 -> [w343] mode=indexing
              n120 = call "Associate a File Extension.vi"("error in (no error)"=w345, "string"=w343, "exe path"=path "") -> ("error out"=w344:errorcluster)  [unwired: 8 in]
            }
          }
        }
      }
      frame "---------- Actions ----------" {
        n121 = call <vilib>:"Add State(s) to Queue__JKI_lib_State_Machine.vi"("State(s) in (\"\")"=w350) -> ("States Out"=w349:string)  [unwired: 14 in]
      }
      frame "Get Opened File Name" {
        n122 = Unbundle By Name(w355) -> ("RuntimeEngine"=w356:bool)
        n123 = case shown="False" w356 {
          tunnel: w362 -> [w364 w372]
          tunnel: [w364 w371] -> w361
          tunnel: ["file path" w370] -> w357
          tunnel: [FALSE w369] -> w354
          frame False {
          }
          frame True {
            n124 = property class="App"(error in=w372) -> (error out=w371:errorcluster, "App.Args"=w368:string[])  [unwired: 1 in, 1 out]
            n125 = Index Array(array=w368) -> (element #2=w367:string)  [unwired: 2 in, 1 out]
            n126 = String To Path(string=w367) -> (path=w370:path)
            n127 = Empty String/Path?(string/path=w370) -> (empty?=w369:bool)
          }
        }
        n128 = Bundle By Name(cluster=w363, "File Path"=w357) -> (w358:refnum<class "application.lvclass">)
        n129 = Select(t="Macro: Enter Setting Mode", s=w354, f="Macro: Enter Normal Mode") -> (s? t:f=w353:string)
        n130 = call <vilib>:"Add State(s) to Queue__JKI_lib_State_Machine.vi"("State(s) in (\"\")"=w359, "State(s) at Back (\"\")"=w353) -> ("States Out"=w360:string)  [unwired: 13 in]
      }
      frame "Find New Symbol" {
        n131 = Unbundle By Name(w376) -> ("File Path"=w382:path)
        n132 = Strip Path(path=w382) -> (stripped path=w381:path)  [unwired: 1 out]
        n133 = call "FindSymbol.vi"("error in (no error)"=w374, "pattern"="DEV ENVIRONMENT *" ("prefix"), "path"=w381) -> ("error out"=w373:errorcluster, "Version"=w379:string, "Exits?"=w377:bool, "found path"=w380:path)  [unwired: 4 in, 1 out]
        n134 = Bundle By Name(cluster=w376, "Symbol Path"=w380, "Symbol Version"=w379, "Symbol Found?"=w377) -> (w375:refnum<class "application.lvclass">)
        n135 = call <vilib>:"Add State(s) to Queue__JKI_lib_State_Machine.vi"("State(s) in (\"\")"=w383) -> ("States Out"=w384:string)  [unwired: 14 in]
      }
      frame "Find Old Symbol" {
        n136 = Unbundle By Name(w389) -> ("File Path"=w395:path)
        n137 = Strip Path(path=w395) -> (stripped path=w394:path)  [unwired: 1 out]
        n138 = call "FindSymbol.vi"("error in (no error)"=w387, "pattern"="开发环境 *" ("prefix"), "path"=w394) -> ("error out"=w386:errorcluster, "Version"=w392:string, "Exits?"=w390:bool, "found path"=w393:path)  [unwired: 4 in, 1 out]
        n139 = Bundle By Name(cluster=w389, "Symbol Path"=w393, "Symbol Version"=w392, "Symbol Found?"=w390) -> (w388:refnum<class "application.lvclass">)
        n140 = call <vilib>:"Add State(s) to Queue__JKI_lib_State_Machine.vi"("State(s) in (\"\")"=w396) -> ("States Out"=w397:string)  [unwired: 14 in]
      }
      frame "Replace with New Symbol" {
        n141 = Unbundle By Name(w401) -> ("Symbol Version"=w403:string, "Symbol Path"=w407:path)
        n142 = call "DeleteSymbolsInDir.vi"("error in (no error)"=w400, "pattern"="开发环境 *", "dup path"=w407) -> ("error in (no error) (dup)"=w405:errorcluster, "dup path (dup)"=w404:path)  [unwired: 7 in]
        n143 = call "CreateSymbolInDir.vi"("error in"=w405, "prefix"="DEV ENVIRONMENT", "Name"=w403, "Path"=w404) -> ("error out"=w399:errorcluster)  [unwired: 6 in, 1 out]
        n144 = call <vilib>:"Add State(s) to Queue__JKI_lib_State_Machine.vi"("State(s) in (\"\")"=w408) -> ("States Out"=w409:string)  [unwired: 14 in]
      }
      frame "Check If The Symbol Version Exist" {
        n145 = Unbundle By Name(w412) -> ("Symbol Found?"=w415:bool, "Version List"=w413:string[], "Symbol Version"=w414:string)
        n146 = case shown="True" w415 {
          tunnel: w413 -> [_ w425]
          tunnel: w414 -> [_ w421]
          tunnel: w412 -> [w420 w423]
          tunnel: [w420 w422] -> w411
          frame False {
          }
          frame True {
            n147 = Search 1D Array(1D array=w425, element=w421) -> (index of element=w426:i32)  [unwired: 1 in]
            n148 = Less Than 0?(x=w426) -> (x < 0?=w424:bool)
            n149 = case shown="True" w424 {
              frame False {
              }
              frame True {
                n150 = One Button Dialog(message="The Symbol Version does not exist on this computer.") -> ()  [unwired: 1 in, 1 out]
              }
            }
            n151 = Bundle By Name(cluster=w423, "Selected Version"=w421) -> (w422:refnum<class "application.lvclass">)
          }
        }
        n152 = call <vilib>:"Add State(s) to Queue__JKI_lib_State_Machine.vi"("State(s) in (\"\")"=w417) -> ("States Out"=w418:string)  [unwired: 14 in]
      }
    }
  }
